vi "Queue.Enqueue.vi"(8 "error in (no error)":errorcluster, 9 "data":variant, 10 "message":string, 11 "queueName":string) -> (0 "error out":errorcluster)   [LabVIEW 2019]
uses:
  QueueMessage.ctl
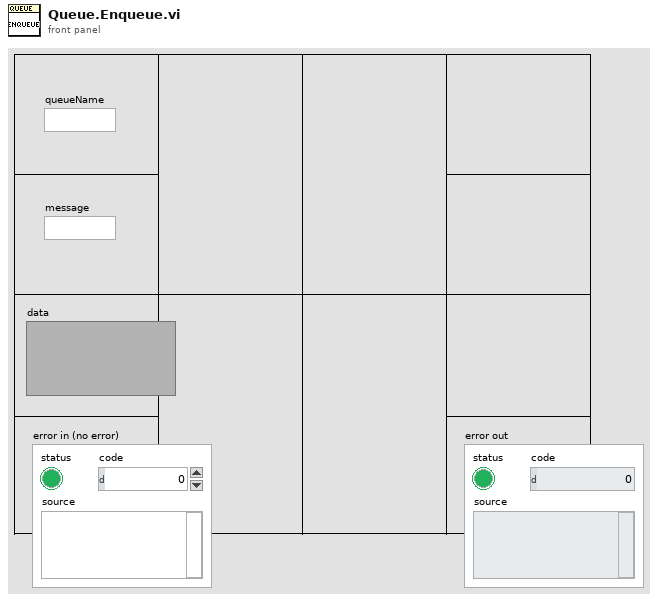
[diagram p1: front panel]
types:
  T1 = typedef "QueueMessage.ctl" = cluster{"message":string, "data":variant}
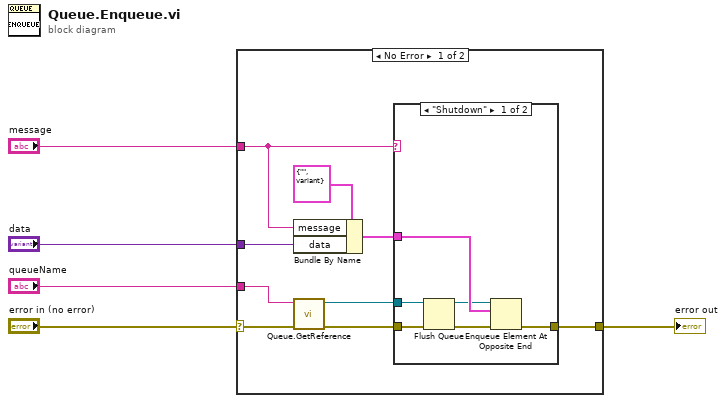
[diagram p0: block diagram]
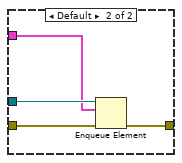
[diagram p2: hidden frame]
diagram:
  n1 = case shown="No Error" "error in (no error)" {
    selector: "error in (no error)" -> [w6 w25]
    tunnel: [w14 w25] -> w1
    tunnel: "queueName" -> [w12 _]
    tunnel: "message" -> [w10 _]
    tunnel: "data" -> [w11 _]
    frame No Error {
      n2 = Bundle By Name(cluster=T1 {"message"="", "data"=variant} ("QueueMessage"), "message"=w10, "data"=w11) -> (w9:T1)
      n3 = call "Queue.GetReference.vi"("error in (no error)"=w6, "queueName"=w12) -> ("error out"=w13:errorcluster, "refToQueue"=w8:refnum<queue>)  [unwired: 8 in]
      n4 = case shown="\"Shutdown\"" w10 {
        tunnel: w13 -> [w17 w24]
        tunnel: [w20 w23] -> w14
        tunnel: w9 -> [w19 w21]
        tunnel: w8 -> [w18 w22]
        frame "Shutdown" {
          n5 = Flush Queue(queue=w18, error in (no error)=w17) -> (queue out=w16:refnum<queue>, error out=w15:errorcluster)  [unwired: 1 out]
          n6 = Enqueue Element At Opposite End(queue=w16, element=w19, error in (no error)=w15) -> (error out=w20:errorcluster)  [unwired: 1 in, 2 out]
        }
        frame Default {
          n7 = Enqueue Element(queue=w22, element=w21, error in (no error)=w24) -> (error out=w23:errorcluster)  [unwired: 1 in, 2 out]
        }
      }
    }
    frame Error {
    }
  }
  "error out" <- w1
